vi "Query_BD.vi"(8 "error in (no error)":errorcluster, 10 "BD":string="BD\\Parametros.db", 11 "Query":string) -> (0 "error out":errorcluster, 3 "Resultado":string[][](array[string]))   [LabVIEW 2019, in "Base de Datos.lvclass"]
doc: "Ejecuta una query en la BD"
uses:
  Base de Datos.lvclass
  SQLiteConnector/SQLiteConnection.lvclass
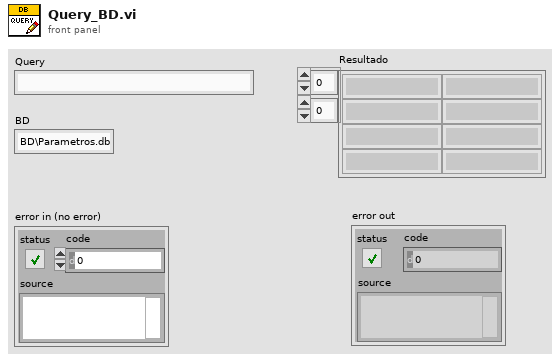
[diagram p1: front panel]
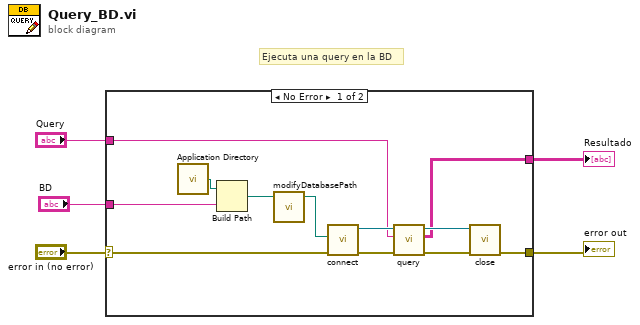
[diagram p0: block diagram]
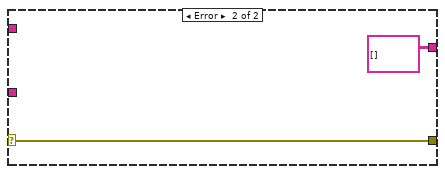
[diagram p2: hidden frame]
diagram:
  # "Ejecuta una query en la BD"
  n1 = case shown="No Error" "error in (no error)" {
    selector: "error in (no error)" -> [w10 w19]
    tunnel: "BD" -> [w8 _]
    tunnel: [w12 w19] -> w4
    tunnel: "Query" -> [w11 _]
    tunnel: [w9 string[][] [] ("result")] -> w1
    frame No Error {
      n2 = call <vilib>:"Application Directory.vi"() -> ("Application Directory"=w16:path)
      n3 = Build Path(base path=w16, name or relative path=w8) -> (appended path=w7:path)
      n4 = call "modifyDatabasePath.vi"("Database Path In"=w7) -> ("Database Path Out"=w6:path)  [unwired: 4 in]
      n5 = call "connect.vi"("error in (no error)"=w10, "Database Path"=w6) -> ("error out"=w15:errorcluster, "object out"=w17:refnum<class "SQLiteConnection.lvclass">)  [unwired: 8 in]
      n6 = call "query.vi"("error in (no error)"=w15, "SQL Statement"=w11, "object in"=w17) -> ("error out"=w14:errorcluster, "result"=w9:string[][], "object out"=w13:refnum<class "SQLiteConnection.lvclass">)  [unwired: 5 in, 1 out]
      n7 = call-dynamic "close.vi"("error in (no error)"=w14, "object in"=w13) -> ("error out"=w12:errorcluster)  [unwired: 8 in, 1 out]
    }
    frame Error {
    }
  }
  "error out" <- w4
  "Resultado" <- w1
